vi "Instrument New Call.vi"(3 "Error In":errorcluster, 4 "Instrument Prop In":T1={"Public"={"Column Name"=[], "Trace Color"=[]}, "Private"={"Path"=path "", "VI Refnum"=refnum, "Name"="", "# of Values"=0, "Scale Factors"=[], "Display"=[], "Offset"=[1.0]}} {"Private"."Offset" format="%^_3e"; "Private"."Scale Factors" format="%^_3e"}, 5 "VI Refnum":T4) -> (0 "Error Out":errorcluster, 1 "Instrument Prop Out":T1={"Public"={"Column Name"=[], "Trace Color"=[]}, "Private"={"Path"=path "", "VI Refnum"=refnum, "Name"="", "# of Values"=0, "Scale Factors"=[], "Display"=[], "Offset"=[1.0]}} {"Private"."Offset" format="%^_3e"; "Private"."Scale Factors" format="%^_3e"})   [LabVIEW 2020]
uses:
  Sub Controls/Instrument Ref.ctl
  Sub Controls/Instrument Properties.ctl
  Sub Controls/Public.ctl
  Sub Controls/Private.ctl
  Sub Controls/SystemCheckBox-resize.ctl
  Sub Controls/Instrument Actions.ctl
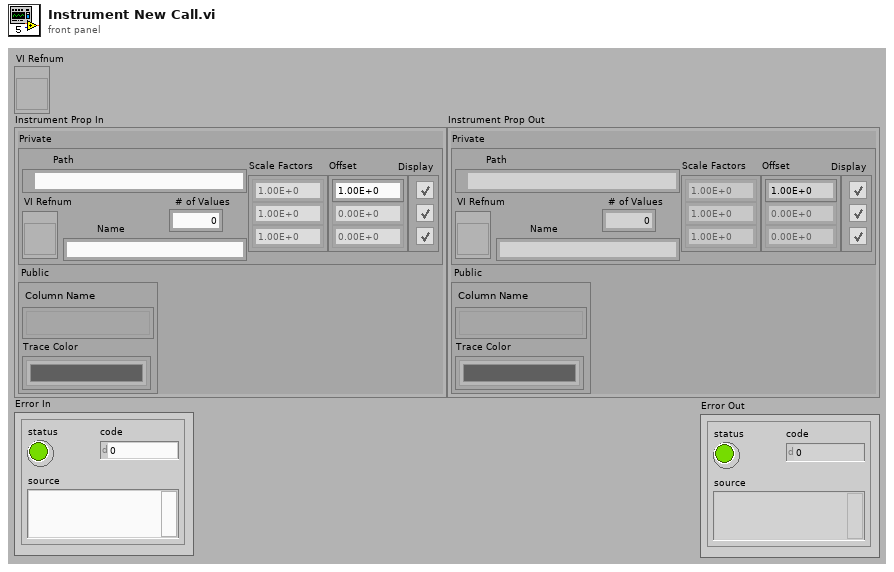
[diagram p1: front panel]
types:
  T1 = typedef "Instrument Properties.ctl" = cluster{"Public":T2, "Private":T3}
  T2 = typedef "Public.ctl" = cluster{"Column Name":string[], "Trace Color":u32[]}
  T3 = typedef "Private.ctl" = cluster{"Path":path, "VI Refnum":T4, "Name":string, "# of Values":i32, "Scale Factors":dbl[], "Display":T5[], "Offset":dbl[]}
  T4 = typedef "Instrument Ref.ctl" = refnum<vi>
  T5 = typedef "SystemCheckBox-resize.ctl" = bool
  T6 = typedef "Instrument Actions.ctl" = enum16{"Scan", "Identify", "New", "Configure", "Initialize", "Test", "Read", "Close"}
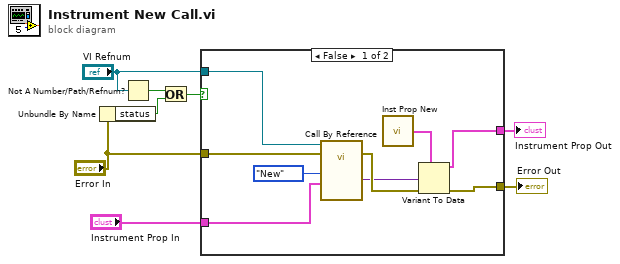
[diagram p0: block diagram]
diagram:
  n1 = Unbundle By Name("Error In") -> ("status"=w1:bool)
  n2 = Not A Number/Path/Refnum?(number/path/refnum="VI Refnum") -> (NaN/Path/Refnum?=w8:bool)
  n3 = Or(x=w8, y=w1) -> (x .or. y?=w2:bool)
  n4 = case shown="False" w2 {
    tunnel: "Error In" -> [w17 w18]
    tunnel: "VI Refnum" -> [w15 _]
    tunnel: [w11 w19] -> w6
    tunnel: [w10 w18] -> w5
    tunnel: "Instrument Prop In" -> [w9 w19]
    frame False {
      n5 = call-by-ref "?"(reference=w15, error in=w17, "Action"=Instrument_Actions."New", "Parameters"=w9) -> (error out=w14:errorcluster, "Output"=w13:variant)  [unwired: 4 in, 2 out]
      n6 = call "Inst Prop New.vi"() -> ("Instrument Prop Out"=w12:T1)
      n7 = Variant To Data(error in=w14, type=w12, Variant=w13) -> (data=w11:T1, error out=w10:errorcluster)
    }
    frame True {
    }
  }
  "Error Out" <- w5
  "Instrument Prop Out" <- w6
